vi "AOI config.vi"(7 "Camera parameters.Id":i32, 8 "error in (no error)":errorcluster, 9 "Caller Enqueuer":refnum<class "Message Enqueuer.lvclass">, 10 "AOI":i32[](array[numeric]), 11 "IMAQdx in":T1) -> (0 "error out":errorcluster, 3 "IMAQdx out":T1)   [LabVIEW 2019, in "Image Acquisition.lvlib" / "Image Acquisition.lvclass"]
uses:
  Image Acquisition.lvclass
  <resource>/objmgr/imaqdx.rc
  <vilib>/userdefined/High Color/IMAQdx.ctl
  <vilib>/ActorFramework/Message Enqueuer/Message Enqueuer.lvclass
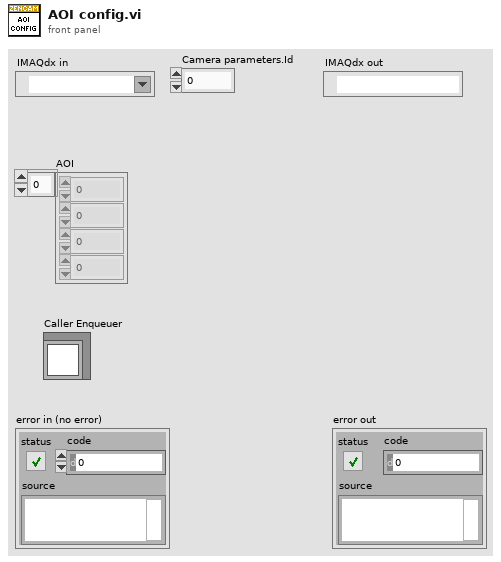
[diagram p1: front panel]
types:
  T1 = typedef "IMAQdx.ctl" = refnum<k21>
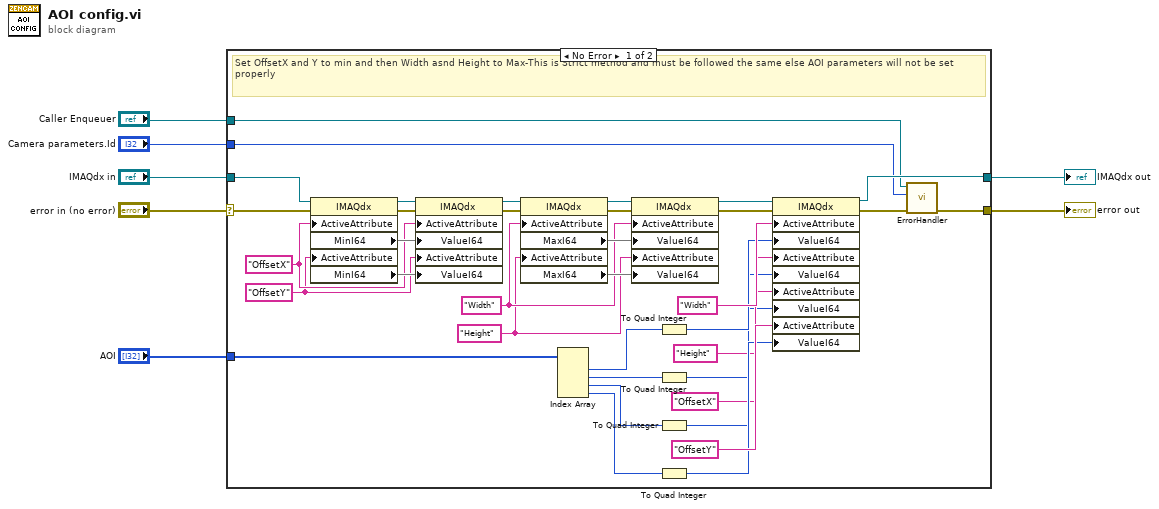
[diagram p0: block diagram]
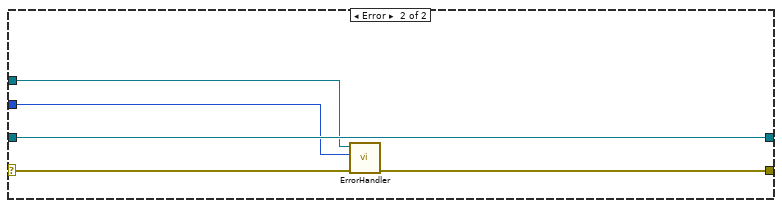
[diagram p2: hidden frame]
diagram:
  n1 = case shown="No Error" "error in (no error)" {
    selector: "error in (no error)" -> [w13 w47]
    tunnel: "IMAQdx in" -> [w14 w48]
    tunnel: [w10 w46] -> w6
    tunnel: [w12 w48] -> w5
    tunnel: "AOI" -> [w25 _]
    tunnel: "Camera parameters.Id" -> [w9 w45]
    tunnel: "Caller Enqueuer" -> [w8 w44]
    frame No Error {
      w29 = "OffsetY" ("ActiveAttribute")
      w30 = "OffsetX" ("ActiveAttribute")
      w27 = "Height" ("ActiveAttribute")
      w28 = "Width" ("ActiveAttribute")
      # "Set OffsetX and Y to min and then Width asnd Height to Max-This is Strict method and must be followed the same else AOI parameters will not be set properly"
      n2 = property class="IMAQdx"(reference=w14, error in=w13, "ActiveAttribute"=w30, "ActiveAttribute"=w29) -> (reference out=w40:T1, error out=w42:errorcluster, "MinI64"=w37, "MinI64"=w38)
      n3 = property class="IMAQdx"(reference=w40, error in=w42, "ActiveAttribute"=w30, "ValueI64"=w37, "ActiveAttribute"=w29, "ValueI64"=w38) -> (reference out=w41:T1, error out=w43:errorcluster)
      n4 = property class="IMAQdx"(reference=w41, error in=w43, "ActiveAttribute"=w28, "ActiveAttribute"=w27) -> (reference out=w32:T1, error out=w35:errorcluster, "MaxI64"=w36, "MaxI64"=w39)
      n5 = Index Array(array=w25) -> (element #1=w24:i32, element #2=w22:i32, element #3=w23:i32, element #4=w21:i32)  [unwired: 4 in]
      n6 = property class="IMAQdx"(reference=w32, error in=w35, "ActiveAttribute"=w28, "ValueI64"=w36, "ActiveAttribute"=w27, "ValueI64"=w39) -> (reference out=w33:T1, error out=w34:errorcluster)
      n7 = To Quad Integer(1:w24) -> (0:w20:i64)
      n8 = To Quad Integer(1:w22) -> (0:w17:i64)
      n9 = To Quad Integer(1:w23) -> (0:w15:i64)
      n10 = To Quad Integer(1:w21) -> (0:w19:i64)
      n11 = property class="IMAQdx"(reference=w33, error in=w34, "ActiveAttribute"="Width", "ValueI64"=w20, "ActiveAttribute"="Height", "ValueI64"=w17, "ActiveAttribute"="OffsetX", "ValueI64"=w15, "ActiveAttribute"="OffsetY", "ValueI64"=w19) -> (reference out=w12:T1, error out=w11:errorcluster)
      n12 = call "ErrorHandler.vi"("error in"=w11, "CameraID"=w9, "Caller Enqueuer"=w8) -> ("error out"=w10:errorcluster)  [unwired: 7 in, 1 out]
    }
    frame Error {
      n13 = call "ErrorHandler.vi"("error in"=w47, "CameraID"=w45, "Caller Enqueuer"=w44) -> ("error out"=w46:errorcluster)  [unwired: 7 in, 1 out]
    }
  }
  "error out" <- w6
  "IMAQdx out" <- w5
